vi "GT Enable Enc Response Check.vi"(8 "error in (no error)":errorcluster caption="错误输入（无错误）", 10 "control":i16, 11 "cardNum":i16) -> (0 "error out":errorcluster caption="错误输出", 3 "function return":i16)   [LabVIEW 2014, in "gts.lvlib"]
doc: "GT_API GT_EnableEncResponseCheck(short cardNum,short control);"
uses:
  gts.lvlib
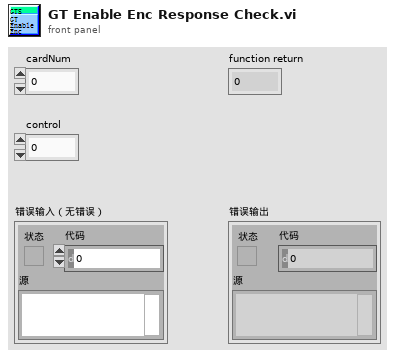
[diagram p1: front panel]
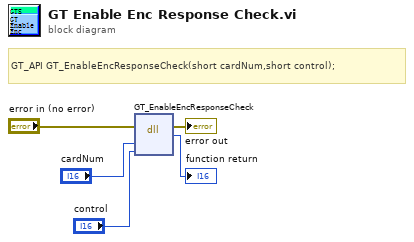
[diagram p0: block diagram]
diagram:
  # "GT_API GT_EnableEncResponseCheck(short cardNum,short control);"
  n1 = dll-call lib="PTH2habs D固高科技资料GTS控制卡GTS卡18年上半年资料dllVC32bit\nmulti_cardgts.*" fn="GT_EnableEncResponseCheck"(error in="error in (no error)", "cardNum"="cardNum", "control"="control") -> (error out=→"error out":errorcluster, →"function return":i16)  [unwired: 4 in, 1 out]
